vi "LabS5_Probe1.vi"() -> ()   [LabVIEW 2012]
uses:
  <vilib>/Analysis/baseanly.llb/Real Dot Product.vi
  <vilib>/Analysis/NI_AALBase.lvlib
panel:
  out "Chart Signal":cluster{"X * Y":dbl, "X * Y":dbl}(graph)
  out "W(k+1)":dbl[](array[numeric])
  out "Chart Error":dbl(graph)
  in  "alpha":dbl
  in  "b":dbl[](array[numeric])
  in  "Offset":dbl
  in  "A":dbl
  out "T":dbl
  in  "Fcon":dbl(knob)=3.229536374351221 scale=1.0..20.0
  in  "Fs":dbl
  in  "Tfinal":dbl
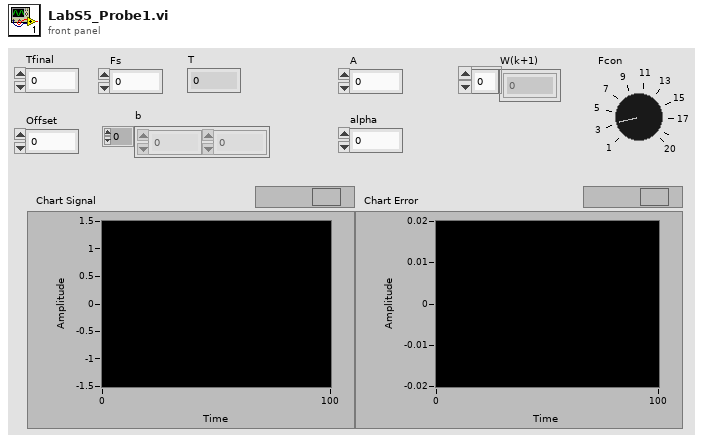
[diagram p1: front panel]
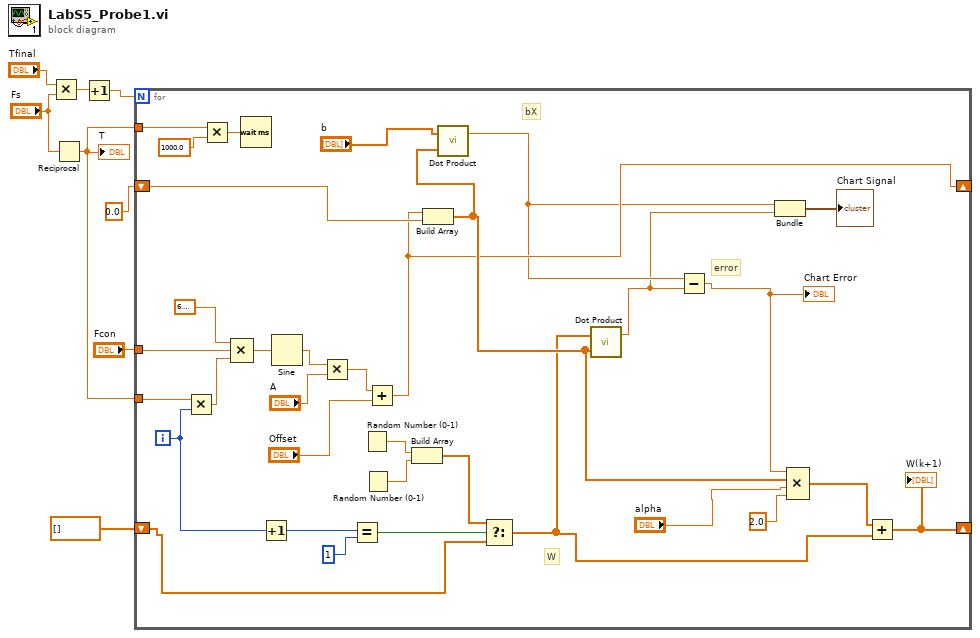
[diagram p0: block diagram]
diagram:
  n1 = Multiply(x="Tfinal", y="Fs") -> (x*y=w7:dbl)
  n2 = Reciprocal(x="Fs") -> (1/x=w1:dbl)
  "T" <- w1
  n3 = Increment(x=w7) -> (x+1=w6:dbl)
  n4 = for {
    N: w6 -> [_]
    tunnel: w1 -> [w39]
    tunnel: "Fcon" -> [w40]
    shift-right: [w17] -> _
    shift-left: 0.0 ("element") -> [w24]
    shift-right: [w18] -> _
    shift-left: dbl[] [] -> [w13]
    tunnel: w1 -> [w11]
    i -> [w31]
    # "W"
    # "bX"
    # "error"
    n5 = Multiply(x=w39, y=w31) -> (x*y=w38:dbl)
    n6 = Multiply(x=w11, y=1000.0) -> (x*y=w12:dbl)
    n7 = Compound Arithmetic op=MULTIPLY(6.283185307179586, w40, w38) -> (w37:dbl)
    n8 = Wait (ms)(milliseconds to wait=w12) -> ()  [unwired: 1 out]
    n9 = Increment(x=w31) -> (x+1=w30:i32)
    n10 = Sine(x=w37) -> (sin(x)=w36:dbl)
    n11 = Multiply(x=w36, y="A") -> (x*y=w34:dbl)
    n12 = Equal?(x=w30, y=1) -> (x = y?=w28:bool)
    n13 = Random Number (0-1)() -> (number: 0 to 1=w27:dbl)
    n14 = Random Number (0-1)() -> (number: 0 to 1=w26:dbl)
    n15 = Add(x=w34, y="Offset") -> (x+y=w17:dbl)
    n16 = Build Array(w27, w26) -> (w25:dbl[])
    n17 = Build Array(w17, w24) -> (w23:dbl[])
    n18 = call-poly <vilib>:"Dot Product.vi"("Y Vector"=w23, "X Vector"="b") -> ("X * Y"=w16:dbl)  [unwired: 1 out]
    n19 = Select(t=w25, s=w28, f=w13) -> (s? t:f=w20:dbl[])
    n20 = call-poly <vilib>:"Dot Product.vi"("Y Vector"=w23, "X Vector"=w20) -> ("X * Y"=w15:dbl)  [unwired: 1 out]
    n21 = Subtract(x=w16, y=w15) -> (x-y=w14:dbl)
    "Chart Error" <- w14
    n22 = Bundle("X * Y"=w16, "X * Y"=w15) -> (→"Chart Signal":cluster{"X * Y":dbl, "X * Y":dbl})  [unwired: 1 in]
    n23 = Compound Arithmetic op=MULTIPLY(w14, w23, "alpha", 2.0 ("value")) -> (w19:dbl[])
    n24 = Add(x=w19, y=w20) -> (x+y=w18:dbl[])
    "W(k+1)" <- w18
  }
